vi "GenerateTestDataFlow.vi"(8 "error in (no error)":errorcluster) -> (0 "Error Out":errorcluster)   [LabVIEW 2017]
uses:
  <vilib>/addons/InsightCM/Utilities/GlobalConfiguration/GlobalConfiguration.lvlib
  <vilib>/addons/PointValueMap/PointValueMap.lvlib
  <vilib>/addons/PointValueMap/subVIs/Point_Read_variant.vi
  <vilib>/addons/PointValueMap/subVIs/Point_Write_variant.vi
  <vilib>/addons/InsightCM/Devices/Shared/DataFlow/controls/DataFlow.ctl
  <vilib>/addons/InsightCM/Devices/Shared/Common/DataFlow/test/SpeedBenchmark/Loop1/Loop1.lvlib
  <vilib>/addons/InsightCM/Devices/Shared/Common/DataFlow/test/SpeedBenchmark/Loop2/Loop2.lvlib
  <vilib>/addons/InsightCM/Devices/Shared/Common/DataFlow/test/SpeedBenchmark/Loop3/Loop3.lvlib
  <vilib>/addons/InsightCM/Devices/Shared/Common/DataFlow/test/SpeedBenchmark/Loop4/Loop4.lvlib
  <vilib>/addons/InsightCM/Devices/Shared/Common/DataFlow/test/SpeedBenchmark/Loop5/Loop5.lvlib
  <vilib>/addons/InsightCM/Devices/Shared/Common/DataFlow/test/SpeedBenchmark/Loop6/Loop6.lvlib
  <vilib>/addons/InsightCM/Devices/Shared/Common/DataFlow/test/SpeedBenchmark/Loop7/Loop7.lvlib
  <vilib>/addons/InsightCM/Devices/Shared/Common/DataFlow/test/SpeedBenchmark/Loop8/Loop8.lvlib
  <vilib>/addons/InsightCM/Devices/Shared/Common/DataFlow/test/SpeedBenchmark/Loop9/Loop9.lvlib
  <vilib>/addons/InsightCM/Devices/Shared/Common/DataFlow/test/SpeedBenchmark/Loop10/Loop10.lvlib
panel:
  out "DataFlow":T1[](array[typedef])
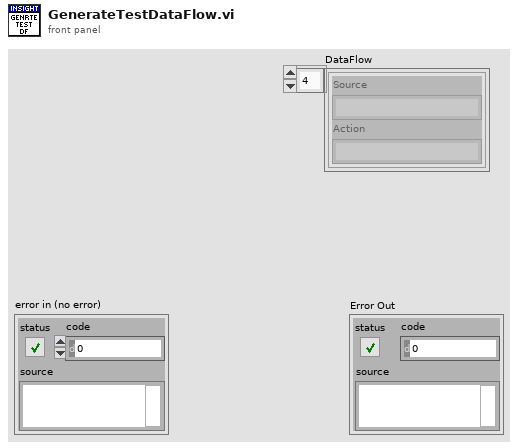
[diagram p1: front panel]
types:
  T1 = typedef "DataFlow.lvlib/DataFlow.ctl" = cluster{"Source":string, "Action":string}
  T2 = typedef "PointValueMap.lvlib/PointMap.ctl" = refnum<data-value>
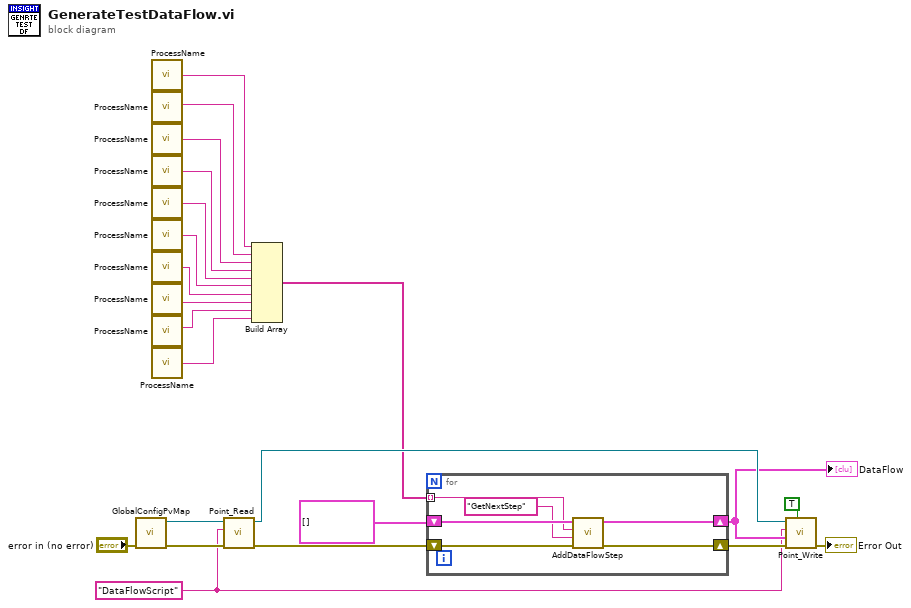
[diagram p0: block diagram]
diagram:
  w11 = "DataFlowScript" ("Name")
  n1 = call <vilib>:"GlobalConfigPvMap.vi"("error in (no error)"="error in (no error)") -> ("error out"=w20:errorcluster, "global configuration map"=w21:T2)  [unwired: 9 in]
  n2 = call <vilib>:"ProcessName.vi"() -> ("ProcessName"=w10:string)  [unwired: 5 in]
  n3 = call <vilib>:"ProcessName.vi"() -> ("ProcessName"=w9:string)  [unwired: 5 in]
  n4 = call <vilib>:"ProcessName.vi"() -> ("ProcessName"=w8:string)  [unwired: 5 in]
  n5 = call <vilib>:"ProcessName.vi"() -> ("ProcessName"=w7:string)  [unwired: 5 in]
  n6 = call <vilib>:"ProcessName.vi"() -> ("ProcessName"=w6:string)  [unwired: 5 in]
  n7 = call <vilib>:"ProcessName.vi"() -> ("ProcessName"=w5:string)  [unwired: 5 in]
  n8 = call <vilib>:"ProcessName.vi"() -> ("ProcessName"=w4:string)  [unwired: 5 in]
  n9 = call <vilib>:"ProcessName.vi"() -> ("ProcessName"=w3:string)  [unwired: 5 in]
  n10 = call <vilib>:"ProcessName.vi"() -> ("ProcessName"=w2:string)  [unwired: 5 in]
  n11 = call <vilib>:"ProcessName.vi"() -> ("ProcessName"=w1:string)  [unwired: 5 in]
  n12 = call-poly <vilib>:"Point_Read.vi"("Error In"=w20, "Tag"=w11, "Map"=w21) -> ("Error Out"=w18:errorcluster, "Map Out"=w15:T2)  [unwired: 3 in, 4 out]
  n13 = Build Array(w10, w9, w8, w7, w6, w5, w4, w3, w2, w1) -> (w13:string[])
  n14 = for {
    shift-right: [w26] -> w12
    shift-left: T1[] [] ("DataFlow") -> [w27]
    shift-right: [w25] -> w16
    shift-left: w18 -> [w28]
    tunnel: w13 -> [w23] mode=indexing
    n15 = call <vilib>:"AddDataFlowStep.vi"("error in (no error)"=w28, "Action"="GetNextStep", "Source"=w23, "DataFlow"=w27) -> ("error out"=w25:errorcluster, "DataFlow"=w26:T1[])  [unwired: 6 in]
  }
  "DataFlow" <- w12
  n16 = call-poly <vilib>:"Point_Write.vi"("Auto Create?"=TRUE, "Error In"=w16, "Value"=w12, "Tag"=w11, "Map"=w15) -> ("Error Out"=→"Error Out":errorcluster)  [unwired: 5 in, 1 out]
